vi "Init_Test.vi"(8 "error in (no error)":errorcluster caption="entrée d'erreur (pas d'erreur)", 11 "Wait_OpenFixture en entrée":refnum<class "Wait_Voltage.lvclass">) -> (0 "error out":errorcluster caption="sortie d'erreur", 3 "Wait_OpenFixture en sortie":refnum<class "Wait_Voltage.lvclass">)   [LabVIEW 2020, in "Library Test.lvlib" / "Wait_Voltage.lvclass"]
uses:
  Wait_Voltage.lvclass
  C:/Users/ngarcin/OneDrive - Altyor/Standard TB/Class/Test/Test (Default)/Test (Default).lvclass
  Commun VI/TypeDef/Commande Test/Commande Type Test.ctl
  Test_Without_Instr/Test_Without_Inst.lvclass
  Instrument/Instrument (Default)/Class Instrument (Default).lvclass
  Wait_Voltage.lvclass/Wait_Voltage.ctl
  Commun VI/Library Commun.lvlib
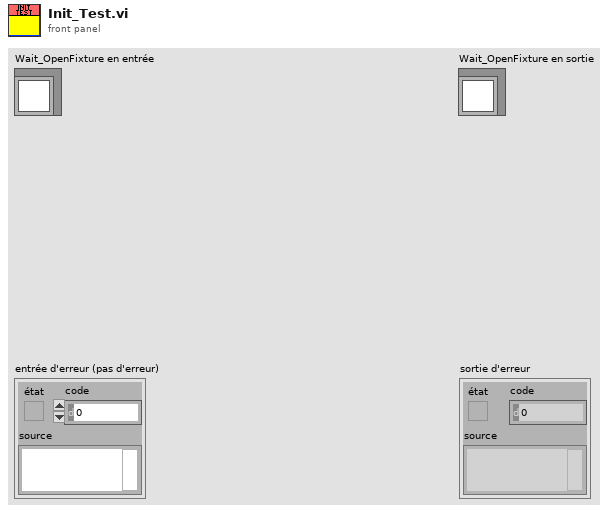
[diagram p1: front panel]
types:
  T1 = typedef "Library Commun.lvlib/Commande Type Test.ctl" = enum16{"Function", "Test", "Calculation"}
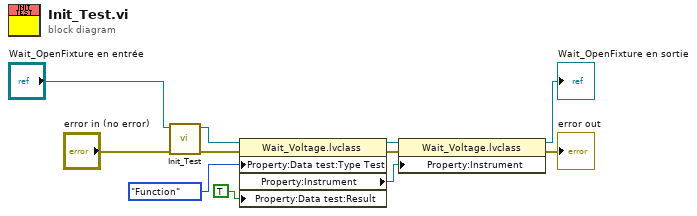
[diagram p0: block diagram]
diagram:
  n1 = call-parent "Init_Test.vi"("error in (no error)"="error in (no error)", "Test_Without_Inst en entrée"="Wait_OpenFixture en entrée") -> ("error out"=w8:errorcluster, "Test_Without_Inst en sortie"=w9:refnum<class "Wait_Voltage.lvclass">)  [unwired: 8 in]
  n2 = property class="Wait_Voltage.lvclass"(reference=w9, error in=w8, "Property:Data test:Type Test"=Commande_Type_Test."Function" ("Type Test"), "Property:Data test:Result"=TRUE ("Result")) -> (reference out=w5:refnum<class "Wait_Voltage.lvclass">, error out=w2:errorcluster, "Property:Instrument"=w1:refnum<class "Class Instrument (Default).lvclass">)
  n3 = property class="Wait_Voltage.lvclass"(reference=w5, error in=w2, "Property:Instrument"=w1) -> (reference out=→"Wait_OpenFixture en sortie":refnum<class "Wait_Voltage.lvclass">, error out=→"error out":errorcluster)
